vi "Result_Test.vi"(8 "error in (no error)":errorcluster caption="entrée d'erreur (pas d'erreur)", 11 "Flash_Jlink en entrée":refnum<class "Get_Mac_Addr.lvclass">) -> (0 "error out":errorcluster caption="sortie d'erreur", 3 "Flash_Jlink en sortie":refnum<class "Get_Mac_Addr.lvclass">)   [LabVIEW 2020, in "Library Test.lvlib" / "Get_Mac_Addr.lvclass"]
uses:
  Get_Mac_Addr.lvclass
  C:/Users/ngarcin/OneDrive - Altyor/Standard TB/Suite TB45/Class/Test/Test (Default)/Test (Default).lvclass
  Commun VI/TypeDef/Variable Printable.ctl
  Flash_Commander/Flash_Commander.lvclass
  Commun VI/Library Commun.lvlib
panel:
  out "Return_State_Machine (Json)":string
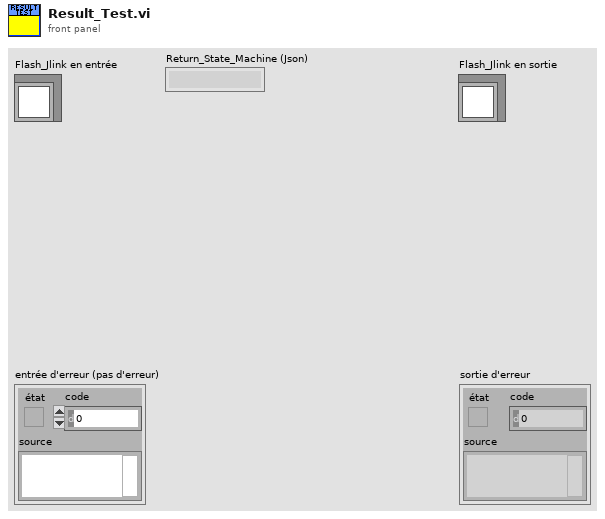
[diagram p1: front panel]
types:
  T1 = typedef "Variable Printable.ctl" = string
  T2 = enum16{"Get Variable", "Get All Variables", "Set Variable", "Delete Variable", "Delete All Variable"}
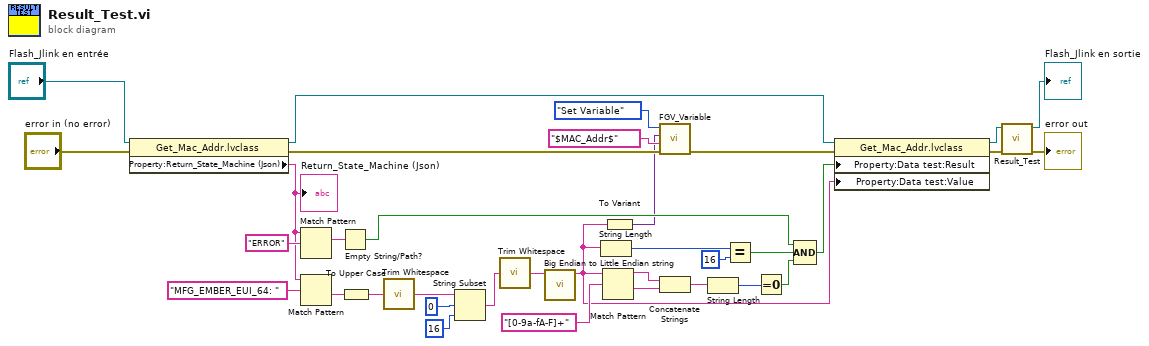
[diagram p0: block diagram]
diagram:
  n1 = property class="Get_Mac_Addr.lvclass"(reference="Flash_Jlink en entrée", error in="error in (no error)") -> (reference out=w17:refnum<class "Get_Mac_Addr.lvclass">, error out=w13:errorcluster, "Property:Return_State_Machine (Json)"=w21:string)
  "Return_State_Machine (Json)" <- w21
  n2 = Match Pattern(string=w21, regular expression="ERROR" ("expression régulière")) -> (match substring=w35:string)  [unwired: 1 in, 3 out]
  n3 = Match Pattern(string=w21, regular expression="MFG_EMBER_EUI_64: ") -> (after substring=w11:string)  [unwired: 1 in, 3 out]
  n4 = Empty String/Path?(string/path=w35) -> (empty?=w20:bool)
  n5 = To Upper Case(1:w11) -> (0:w33:string)
  n6 = call <vilib>:"Trim Whitespace.vi"("string"=w33) -> ("trimmed string"=w29:string)  [unwired: 1 in]
  n7 = String Subset(string=w29, offset (0)=0 ("length (rest)"), length (rest)=16 ("length (rest)")) -> (substring=w9:string)
  n8 = call <vilib>:"Trim Whitespace.vi"("string"=w9) -> ("trimmed string"=w8:string)  [unwired: 1 in]
  n9 = call "Big Endian to Little Endian string.vi"("Input (Big Endian)"=w8) -> ("Output (Little Endian)"=w7:string)  [unwired: 10 in]
  n10 = String Length(string=w7) -> (length=w22:i32)
  n11 = Match Pattern(string=w7, regular expression="[0-9a-fA-F]+") -> (before substring=w23:string, after substring=w24:string)  [unwired: 1 in, 2 out]
  n12 = To Variant(anything=w7) -> (Variant=w10:variant)
  n13 = call "FGV_Variable.vi"("error in (no error)"=w13, "Variable"=T1 "$MAC_Addr$" ("Variable Printable"), "Data In"=w10, "Function"=T2."Set Variable") -> ("error out"=w12:errorcluster)  [unwired: 5 in, 2 out]
  n14 = Concatenate Strings(w23, w24) -> (w25:string)
  n15 = String Length(string=w25) -> (length=w26:i32)
  n16 = Equal?(x=w22, y=16) -> (x = y?=w19:bool)
  n17 = Equal To 0?(x=w26) -> (x = 0?=w18:bool)
  n18 = Compound Arithmetic op=AND(w20, w19, w18) -> (w16:bool)
  n19 = property class="Get_Mac_Addr.lvclass"(reference=w17, error in=w12, "Property:Data test:Result"=w16, "Property:Data test:Value"=w7) -> (reference out=w4:refnum<class "Get_Mac_Addr.lvclass">, error out=w6:errorcluster)
  n20 = call-parent "Result_Test.vi"("error in (no error)"=w6, "Flash_Jlink en entrée"=w4) -> ("error out"=→"error out":errorcluster, "Flash_Jlink en sortie"=→"Flash_Jlink en sortie":refnum<class "Get_Mac_Addr.lvclass">)  [unwired: 8 in]
